vi "CSV Open.vi"(9 "2D Array In":dbl[][](array[numeric]), 11 "Open":bool) -> (1 "2D Array Out":dbl[][](array[numeric]))   [LabVIEW 2018]
uses:
  <vilib>/Utility/file.llb/Read From Spreadsheet File (DBL).vi
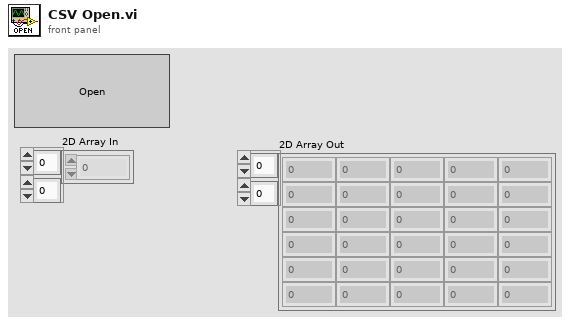
[diagram p1: front panel]
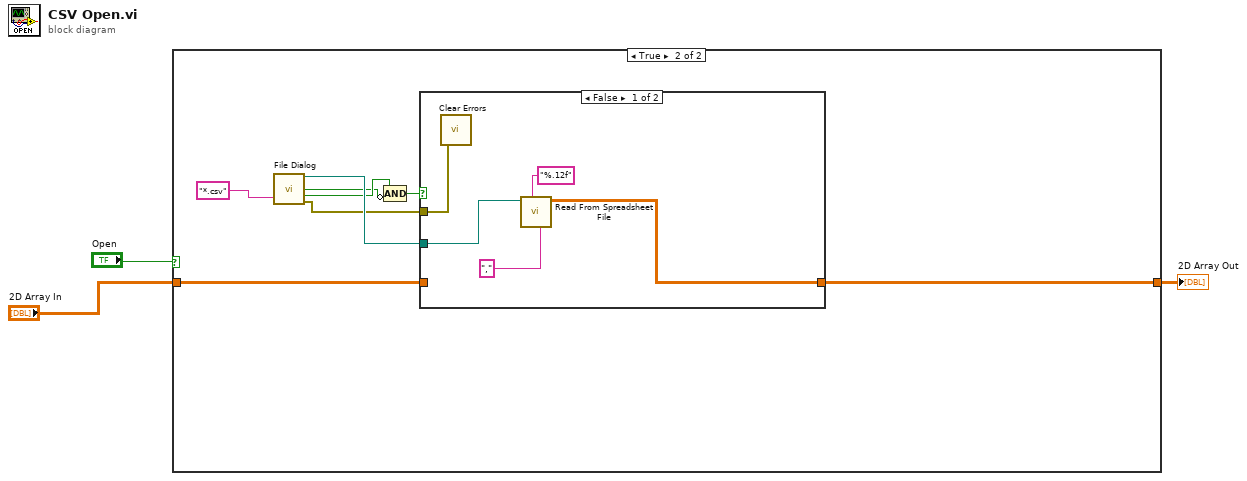
[diagram p0: block diagram]
diagram:
  n1 = case shown="True" "Open" {
    tunnel: [w4 w12] -> w1
    tunnel: "2D Array In" -> [w4 w5]
    frame False {
    }
    frame True {
      n2 = call "File Dialog"("pattern (all files)"="*.csv") -> ("selected path"=w11:path, "exists"=w6:bool, "cancelled"=w7:bool, "error out"=w9:errorcluster)  [unwired: 11 in]
      n3 = Compound Arithmetic op=AND(w7, invert w6) -> (w8:bool)
      n4 = case shown="False" w8 {
        tunnel: w11 -> [w17 _]
        tunnel: [w13 w18] -> w12
        tunnel: w9 -> [w16 _]
        tunnel: w5 -> [_ w18]
        frame False {
          n5 = call <vilib>:"Clear Errors.vi"("error in (no error)"=w16) -> ()  [unwired: 5 in, 2 out]
          n6 = call-poly <vilib>:"Read From Spreadsheet File.vi"("delimiter (\\t)"="," ("delimiter (\\t)"), "format (%.3f)"="%.12f", "file path (dialog if empty)"=w17) -> ("all rows"=w13:dbl[][])  [unwired: 4 in, 4 out]
        }
        frame True {
        }
      }
    }
  }
  "2D Array Out" <- w1
